vi "Stop.vi"(8 "error in (no error)":errorcluster, 11 "Object ref in":T1) -> (0 "error out":errorcluster, 3 "Object ref out":T1)   [LabVIEW 2013, in "SLMControl.lvlib" / "SC-Main.lvclass"]
uses:
  SC-Main.lvclass
  Object-reference.ctl
  SC-Main.lvclass/SC-Main.ctl
  Application-status.ctl
  Deposition-actions.ctl
  Lasing-actions.ctl
  UI/Control-names.ctl
  Read UI.vi
  Read Status.vi
  UI/Set-control-enable-multiple.vi
  UI/Set-control-boolean.vi
  UI/SC-UI.lvclass
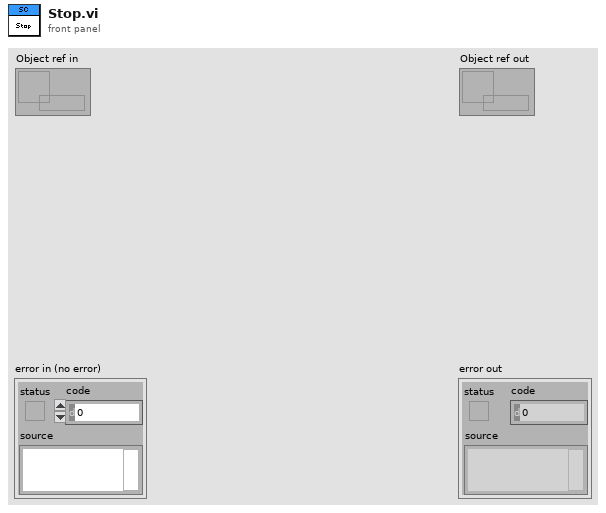
[diagram p1: front panel]
types:
  T1 = typedef "SLMControl.lvlib/SC-Main.lvclass/Object-reference.ctl" = refnum<data-value>
  T2 = typedef "SLMControl.lvlib/SC-UI.lvclass/Control-names.ctl" = enum16{"Com-in", "Com-out", "Help", "Status", "Load configuration", "Save configuration", "Load lasing files", "Load deposition files", "Clear", "Files", "Activate", "Execute", "Abort", "Options", "Current layer", "Current iteration", "Last elapsed time", "Deposition status", "Lasing job", "Status LEDs", "Exiting led", "Initialized led", "Files loaded led", "Activated led", "Executing led", "Deposition led", "Lasing job led", "Lasing led"}
  T3 = typedef "SLMControl.lvlib/SC-Main.lvclass/Lasing-actions.ctl" = enum16{"Idle", "Activate", "Load lasing file", "Launch lasing", "Wait for lasing end", "Signal iterate", "Signal abort", "Abort", "Reset", "Exit"}
  T4 = typedef "SLMControl.lvlib/SC-Main.lvclass/Deposition-actions.ctl" = enum16{"Idle", "Activate", "Load deposition", "Launch deposition", "Wait for deposition end", "Signal lasing", "Abort", "Reset", "Exit"}
  T5 = typedef "SLMControl.lvlib/SC-Main.lvclass/Application-status.ctl" = enum16{"Idle", "Initialized", "Configured", "Activated", "Started", "Paused", "Stopped", "Reset", "Error", "Exited"}
  T6 = typedef "SLMControl.lvlib/SC-Main.lvclass/Client-status.ctl" = enum16{"Idle", "Initialized", "Configured", "Activated", "Started", "Paused", "Stopped", "Reset", "Error", "Exited"}
  T7 = typedef "SLMControl.lvlib/SC-UI.lvclass/Panes-reference.ctl" = refnum<data-value>
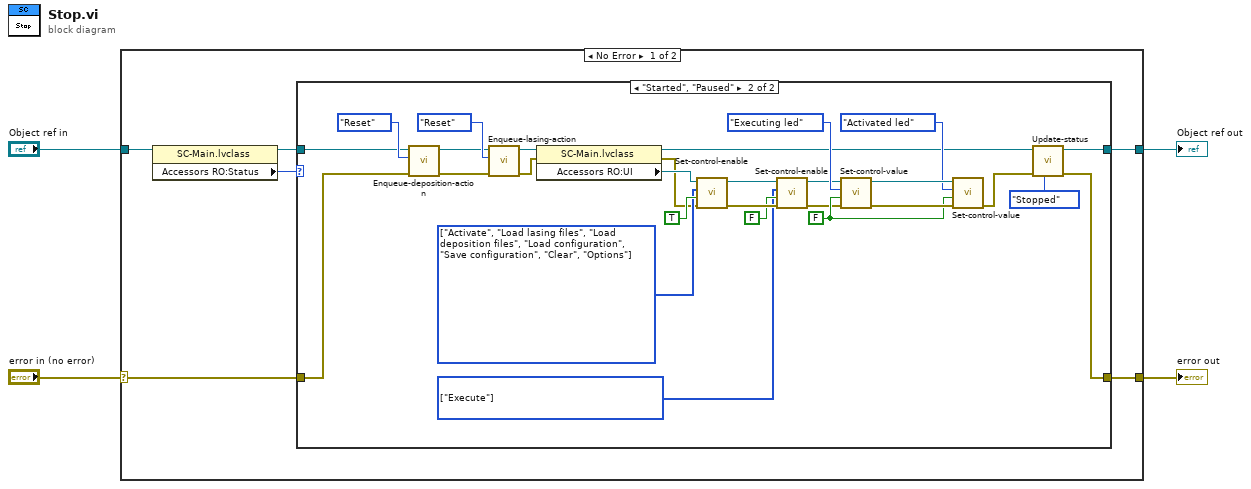
[diagram p0: block diagram]
diagram:
  n1 = case shown="No Error" "error in (no error)" {
    selector: "error in (no error)" -> [w8 w42]
    tunnel: [w10 w42] -> w3
    tunnel: [w9 w41] -> w1
    tunnel: "Object ref in" -> [w7 w41]
    frame No Error {
      n2 = property class="SC-Main.lvclass"(reference=w7) -> (reference out=w6:T1, "Accessors RO:Status"=w5:T6)  [unwired: 1 in, 1 out]
      n3 = case shown="\"Started\", \"Paused\"" w5 {
        tunnel: [w11 w39] -> w10
        tunnel: [w12 w38] -> w9
        tunnel: w6 -> [w12 w13]
        tunnel: w8 -> [w11 w24]
        frame "Idle", Default {
        }
        frame "Started", "Paused" {
          w14 = T2[] [enum."Execute"] items=["Com-in", "Com-out", "Help", "Status", "Load configuration", "Save configuration", "Load lasing files", "Load deposition files", "Clear", "Files", "Activate", "Execute", "Abort", "Options", "Current layer", "Current iteration", "Last elapsed time", "Deposition status", "Lasing job", "Status LEDs", "Exiting led", "Initialized led", "Files loaded led", "Activated led", "Executing led", "Deposition led", "Lasing job led", "Lasing led"] ("Control names")
          w21 = T2[] [enum."Activate", enum."Load lasing files", enum."Load deposition files", enum."Load configuration", enum."Save configuration", enum."Clear", enum."Options"] items=["Com-in", "Com-out", "Help", "Status", "Load configuration", "Save configuration", "Load lasing files", "Load deposition files", "Clear", "Files", "Activate", "Execute", "Abort", "Options", "Current layer", "Current iteration", "Last elapsed time", "Deposition status", "Lasing job", "Status LEDs", "Exiting led", "Initialized led", "Files loaded led", "Activated led", "Executing led", "Deposition led", "Lasing job led", "Lasing led"] ("Control names")
          w25 = FALSE
          n4 = call "Enqueue-deposition-action.vi"("error in (no error)"=w24, "Action"=Deposition-actions."Reset" ("Execution action"), "State queue in"=w13) -> ("error out"=w34:errorcluster, "State queue out"=w35:T1)  [unwired: 6 in, 1 out]
          n5 = call "Enqueue-lasing-action.vi"("error in (no error)"=w34, "Action"=Lasing-actions."Reset" ("Execution action"), "State queue in"=w35) -> ("error out"=w28:errorcluster, "State queue out"=w33:T1)  [unwired: 6 in, 1 out]
          n6 = property class="SC-Main.lvclass"(reference=w33, error in=w28) -> (reference out=w29:T1, error out=w20:errorcluster, "Accessors RO:UI"=w22:T7)
          n7 = call-poly "Set-control-enable.vi"("error in (no error)"=w20, "Enable?"=TRUE, "Control names"=w21, "Panes in"=w22) -> ("error out"=w16:errorcluster, "Panes out"=w19:T7)  [unwired: 6 in]
          n8 = call-poly "Set-control-enable.vi"("error in (no error)"=w16, "Enable?"=FALSE, "Control names"=w14, "Panes in"=w19) -> ("error out"=w17:errorcluster, "Panes out"=w18:T7)  [unwired: 6 in]
          n9 = call-poly "Set-control-value.vi"("error in (no error)"=w17, "Value"=w25, "Control name"=Control-names."Executing led", "Panes in"=w18) -> ("error out"=w27:errorcluster, "Panes out"=w32:T7)  [unwired: 6 in]
          n10 = call-poly "Set-control-value.vi"("error in (no error)"=w27, "Value"=w25, "Control name"=Control-names."Activated led", "Panes in"=w32) -> ("error out"=w26:errorcluster)  [unwired: 6 in, 1 out]
          n11 = call "Update-status.vi"("Status"=Application-status."Stopped", "error in (no error)"=w26, "Object ref in"=w29) -> ("error out"=w39:errorcluster, "Object ref out"=w38:T1)  [unwired: 7 in]
        }
      }
    }
    frame Error {
    }
  }
  "error out" <- w3
  "Object ref out" <- w1
